vi "convert output indicies to typedef data.vi"(8 "error in":errorcluster, 11 "Output Mapping Info":T1) -> (0 "error out":errorcluster, 3 "Outputs to system":T2)   [LabVIEW 2013, in "fixed channel tag bus module.lvclass"]
uses:
  fixed channel tag bus module.lvclass
  outputs.ctl
  <vilib>/NI/Tag Bus Data Framework/Utilities/Cluster to Tag Bus Scripts/Channel Run Time Mapping Info.ctl
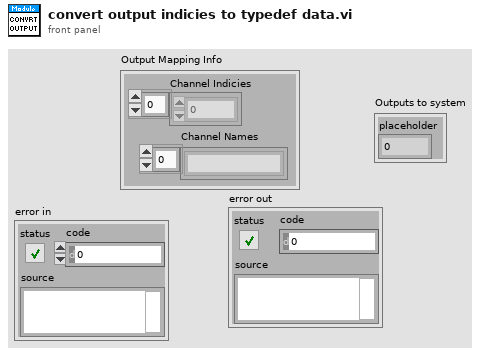
[diagram p1: front panel]
types:
  T1 = typedef "Channel Run Time Mapping Info.ctl" = cluster{"Channel Indicies":i32[], "Channel Names":string[]}
  T2 = typedef "fixed channel tag bus module.lvclass/outputs.ctl" = cluster{"placeholder":i32}
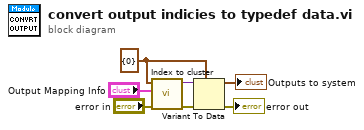
[diagram p0: block diagram]
diagram:
  w4 = T2 {"placeholder"=0} ("Outputs to system")
  n1 = call <vilib>:"Index to cluster.vi"("error in"="error in", "Input Mapping Info"="Output Mapping Info", "Variant in"=w4) -> ("error out"=w7:errorcluster, "Variant out"=w6:variant)  [unwired: 7 in]
  n2 = Variant To Data(error in=w7, type=w4, Variant=w6) -> (data=→"Outputs to system":T2, error out=→"error out":errorcluster)
